vi "Write Base I32.vi"(4 "timestamps":timestamp[](array[numeric]), 6 "index_channel":u32, 8 "error in":errorcluster, 9 "data":i32[][](array[numeric]), 10 "channels":u32[](array[numeric]), 11 "Writer":refnum<class "Synnax Writer.lvclass">) -> (0 "error out":errorcluster, 3 "Writer Out":refnum<class "Synnax Writer.lvclass">)   [LabVIEW 2026, in "synnax_lib.lvlib" / "Synnax Writer.lvclass"]
doc: "SYNNAX_EXPORT int32_t synnax_writer_write(\n SynnaxWriter writer,\n uint32_t channel,\n const double *data,\n uint64_t sample_count,\n SynnaxError err\n);"
uses:
  Synnax Writer.lvclass
  Synnax Writer.lvclass/Synnax Writer.ctl
  <vilib>/Utility/error.llb/Error Cluster From Error Code.vi
  synnax_lib.lvlib
  synnax_clib.dll
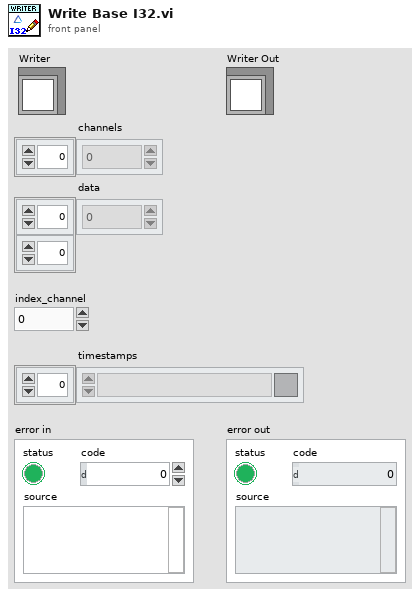
[diagram p1: front panel]
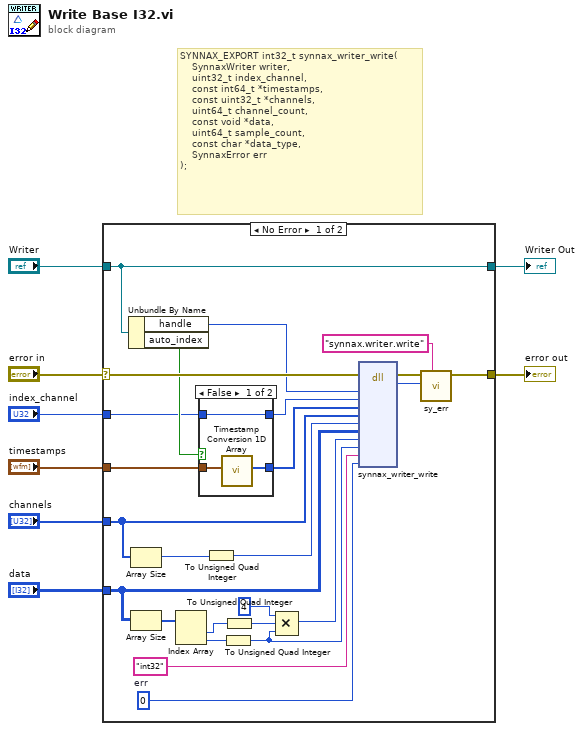
[diagram p0: block diagram]
diagram:
  # "SYNNAX_EXPORT int32_t synnax_writer_write(\n    SynnaxWriter writer,\n    uint32_t index_channel,\n    const int64_t *timestamps,\n    const uint32_t *channels,\n    uint64_t channel_count,\n    const void *data,\n    uint64_t sample_count,\n    const char *data_type,\n    SynnaxError err\n);"
  n1 = case shown="No Error" "error in" {
    selector: "error in" -> [w27 w38]
    tunnel: "index_channel" -> [w22 _]
    tunnel: [w20 w38] -> w7
    tunnel: "channels" -> [w28 _]
    tunnel: "data" -> [w13 _]
    tunnel: "timestamps" -> [w25 _]
    tunnel: "Writer" -> [w19 w37]
    tunnel: [w19 w37] -> w1
    frame No Error {
      w17 = u64 0  # err
      n2 = Unbundle By Name(w19) -> ("handle"=w26:u64, "auto_index"=w23:bool)
      n3 = Array Size(array=w28) -> (size(s)=w30:i32)
      n4 = Array Size(array=w13) -> (size(s)=w12:i32[])
      n5 = Index Array(array=w12) -> (element #1=w15:i32, element #2=w16:i32)  [unwired: 2 in]
      n6 = case shown="False" w23 {
        tunnel: w25 -> [w36 _]
        tunnel: [w35 _] -> w24
        tunnel: [w34 _] -> w21
        tunnel: w22 -> [w34 _]
        frame False {
          n7 = call "Timestamp Conversion 1D Array.vi"("timestamps"=w36) -> ("timestamps (ns)"=w35:i64[])  [unwired: 9 in]
        }
        frame True {
        }
      }
      n8 = To Unsigned Quad Integer(1:w30) -> (0:w29:u64)
      n9 = To Unsigned Quad Integer(1:w16) -> (0:w10:u64)
      n10 = To Unsigned Quad Integer(1:w15) -> (0:w14:u64)
      n11 = Compound Arithmetic op=MULTIPLY(u64 4, w14, w10) -> (w9:u64)
      n12 = dll-call lib="C/synnax/client/lv/synnax_clib.dll" fn="synnax_writer_write"(error in=w27, "writer"=w26, "index_channel"=w21, "timestamps"=w24, "channels"=w28, "channel_count"=w29, "data"=w13, "data_size"=w9, "sample_count"=w10, "data_type"="int32", "err"=w17) -> (error out=w33:errorcluster, "return type"=w32:i32)  [unwired: 12 in, 1 out]
      n13 = call "sy_err.vi"("source"="synnax.writer.write", "error code"=w32, "error in (no error)"=w33) -> ("error out"=w20:errorcluster)  [unwired: 8 in]
    }
    frame Error {
    }
  }
  "error out" <- w7
  "Writer Out" <- w1
